vi "Tx.vi"(0 "tx.parameters":T7={"tx.trigger select"=enum."Software", "tx.trigger enable"=FALSE, "tx.trigger sync enable"=FALSE, "tx 0.stream enable"=FALSE, "tx 1.stream enable"=FALSE, "tx.software trigger"=FALSE, "tx.reset"=FALSE, "tx.abort"=FALSE, "tx.samples to generate"=0, "duc parameters"=[{"frequency shift"=0.0, "impairments"={"inline gain I"=0.0, "inline gain Q"=0.0, "cross gain I"=0.0, "cross gain Q"=0.0, "pre-gain offset I"=0.0, "pre-gain offset Q"=0.0, "post-gain offset I"=0.0, "post-gain offset Q"=0.0}, "phase"=0.0, "input sample rate"=0.0, "gain"={"gain I"=0.0, "gain Q"=0.0}, "delay"=0.0}, {"frequency shift"=0.0, "impairments"={"inline gain I"=0.0, "inline gain Q"=0.0, "cross gain I"=0.0, "cross gain Q"=0.0, "pre-gain offset I"=0.0, "pre-gain offset Q"=0.0, "post-gain offset I"=0.0, "post-gain offset Q"=0.0}, "phase"=0.0, "input sample rate"=0.0, "gain"={"gain I"=0.0, "gain Q"=0.0}, "delay"=0.0}]} {"duc parameters"."frequency shift" format="%#.48g"}, 5 "tx.start trigger":bool) -> (4 "tx.status":T2)   [LabVIEW 2023]
uses:
  <instrlib>/_niInstr/DSP/v1/Shared/Public/IQ Impairments.ctl
  <instrlib>/_niInstr/DSP/v1/Shared/Public/IQ Gain.ctl
  <instrlib>/niUSRP/Reference FPGA/SubVIs/DUC Parameters.ctl
  <instrlib>/niVST/Reference FPGA/FPGA/USRPRIO Sample VIs/Host/SubVIs/Start Trigger.ctl
  <instrlib>/niUSRP/Reference FPGA/SubVIs/Stream Control State.ctl
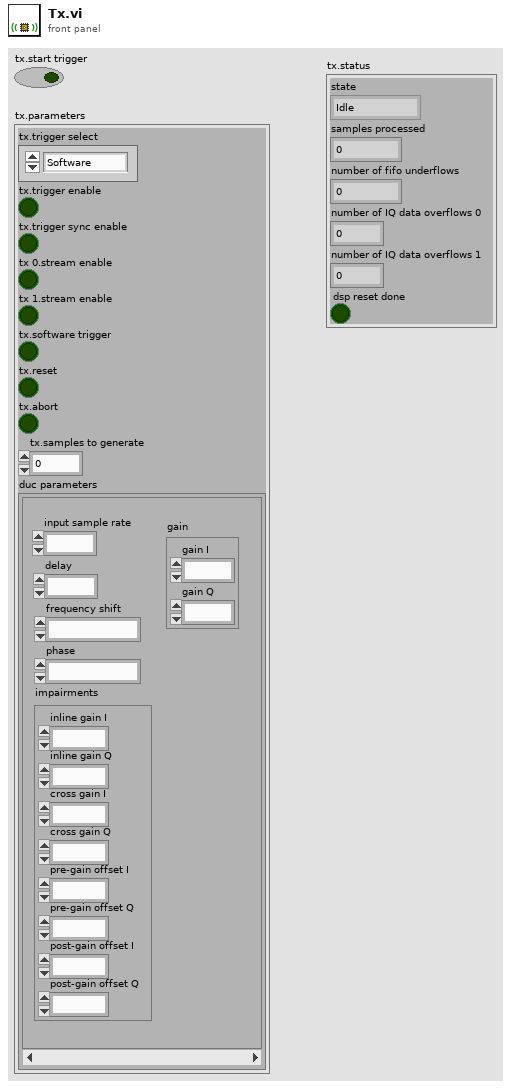
[diagram p1: front panel]
types:
  T1 = typedef "Stream Control State.ctl" = enum16{"Idle", "Active", "WaitForTrigger"}
  T2 = cluster{"state":T1, "samples processed":u32, "number of fifo underflows":u32, "number of IQ data overflows 0":u64, "number of IQ data overflows 1":u64, "dsp reset done":bool}
  T3 = typedef "Start Trigger.ctl" = enum8{"Software", "Digital Edge", "Rx Start Trigger", "Tx Start Trigger", "Immediate", "Future Time Event"}
  T4 = typedef "DUC Parameters.ctl" = cluster{"frequency shift":fxp<+/-,48,0>, "impairments":T5, "phase":fxp<+/-,21,0>, "input sample rate":fxp<+,48,1>, "gain":T6, "delay":fxp<+/-,18,0>}
  T5 = typedef "niInstr DSP v1 Shared.lvlib/IQ Impairments.ctl" = cluster{"inline gain I":fxp<+/-,18,1>, "inline gain Q":fxp<+/-,18,1>, "cross gain I":fxp<+/-,18,1>, "cross gain Q":fxp<+/-,18,1>, "pre-gain offset I":fxp<+/-,18,1>, "pre-gain offset Q":fxp<+/-,18,1>, "post-gain offset I":fxp<+/-,18,1>, "post-gain offset Q":fxp<+/-,18,1>}
  T6 = typedef "niInstr DSP v1 Shared.lvlib/IQ Gain.ctl" = cluster{"gain I":fxp<+/-,24,3>, "gain Q":fxp<+/-,24,3>}
  T7 = cluster{"tx.trigger select":T3, "tx.trigger enable":bool, "tx.trigger sync enable":bool, "tx 0.stream enable":bool, "tx 1.stream enable":bool, "tx.software trigger":bool, "tx.reset":bool, "tx.abort":bool, "tx.samples to generate":u32, "duc parameters":T4[]}
  T8 = cluster{"tx.state":T1, "tx.samples processed":u32, "tx.number of fifo underflows":u32, "tx 0.number of IQ data overflows":u64, "tx 1.number of IQ data overflows":u64, "tx.dsp reset done":bool}
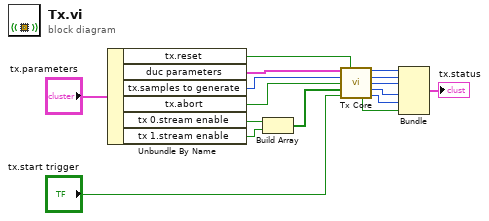
[diagram p0: block diagram]
diagram:
  n1 = Unbundle By Name("tx.parameters") -> ("tx.reset"=w14:bool, "duc parameters"=w15:T4[], "tx.samples to generate"=w13:u32, "tx.abort"=w12:bool, "tx 0.stream enable"=w11:bool, "tx 1.stream enable"=w10:bool)
  n2 = Build Array(w11, w10) -> (w9:bool[])
  n3 = call <instrlib>:"Tx Core.vi"("duc parameters"=w15, "tx.reset"=w14, "tx.samples to generate"=w13, "tx.abort"=w12, "tx.stream enable"=w9, "tx.start trigger"="tx.start trigger") -> ("tx.state"=w7:T1, "tx.samples processed"=w6:u32, "tx.number of fifo underflows"=w5:u32, "tx 0.number of IQ data overflows"=w4:u64, "tx.dsp reset done"=w2:bool, "tx 1.number of IQ data overflows"=w3:u64)  [unwired: 4 in]
  n4 = Bundle("tx.state"=w7, "tx.samples processed"=w6, "tx.number of fifo underflows"=w5, "tx 0.number of IQ data overflows"=w4, "tx 1.number of IQ data overflows"=w3, "tx.dsp reset done"=w2) -> (→"tx.status":T8)  [unwired: 1 in]
